vi "Zip.vi"   [LabVIEW 2020]
panel:
  # "Zip File"
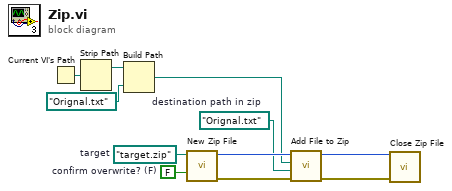
[diagram p0: block diagram]
diagram:
  w5 = FALSE  # confirm overwrite? (F)
  w6 = path "Orignal.txt"  # destination path in zip
  w7 = path "target.zip"  # target
  n1 = Current VI's Path() -> (path=w4:path)
  n2 = Strip Path(path=w4) -> (stripped path=w3:path)  [unwired: 1 out]
  n3 = Build Path(base path=w3, name or relative path=path "Orignal.txt" ("source file path")) -> (appended path=w1:path)
  n4 = call <vilib>:"New Zip File.vi"("confirm overwrite? (F)"=w5, "target"=w7) -> ("error out"=w9:errorcluster, "zip file out"=w11:i64)  [unwired: 3 in, 1 out]
  n5 = call <vilib>:"Add File to Zip.vi"("error in (no error)"=w9, "destination path in zip"=w6, "source file path"=w1, "zip file in"=w11) -> ("error out"=w8:errorcluster, "zip file out"=w10:i64)  [unwired: 6 in]
  n6 = call <vilib>:"Close Zip File.vi"("error in (no error)"=w8, "zip file in"=w10) -> ()  [unwired: 5 in, 1 out]
